vi "udp_vastu.vi"() -> ()   [LabVIEW 2020]
panel:
  out "String":string
  in  "Stop":bool
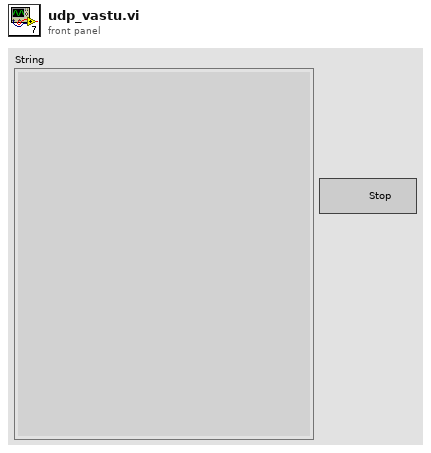
[diagram p1: front panel]
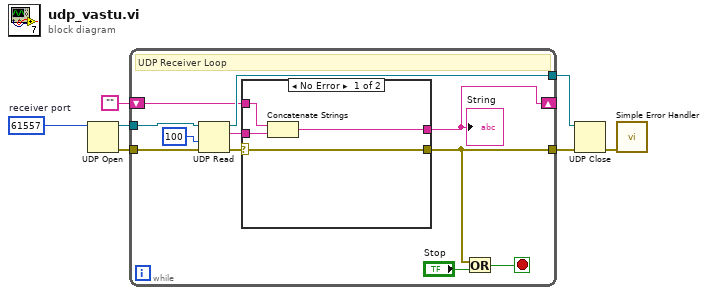
[diagram p0: block diagram]
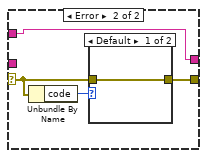
[diagram p2: hidden frame]
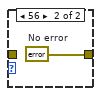
[diagram p3: hidden frame]
diagram:
  w2 = u16 61557  # receiver port
  n1 = UDP Open(11:w2) -> (port=w3:refnum<k16>, 0:w4:errorcluster)  [unwired: 4 in, 1 out]
  n2 = while {
    tunnel: w3 -> [w18]
    tunnel: [w10] -> w7
    tunnel: w4 -> [w15]
    tunnel: [w11] -> w5
    shift-right: [w8] -> _
    shift-left: "" -> [w9]
    stop <- w16 stop-if-true
    # "UDP Receiver Loop"
    n3 = UDP Read(connection ID=w18, timeout ms (25000)=100, 8:w15) -> (data out=w13:string, error out=w12:errorcluster, 3:w10:refnum<k16>)  [unwired: 3 out]
    n4 = case shown="No Error" w12 {
      selector: w12 -> [w22 w25]
      tunnel: w13 -> [w21 _]
      tunnel: [w22 w24] -> w11
      tunnel: w9 -> [w20 w23]
      tunnel: [w19 w23] -> w8
      frame No Error {
        # "Sender sent data. Update chat."
        n5 = Concatenate Strings(w20, w21) -> (w19:string)
      }
      frame Error {
        # "Sender did not send data. Ignore timeout error and keep waiting."
        n6 = Unbundle By Name(w25) -> ("code"=w26:i32)
        n7 = case shown="Default" w26 {
          tunnel: w25 -> [w27 _]
          tunnel: [w27 w28] -> w24
          frame Default {
          }
          frame 56 {
            w28 = errorcluster {"status"=FALSE, "code"=0, "source"=""}  # No error
          }
        }
      }
    }
    "String" <- w8
    n8 = Or(x=w11, y="Stop") -> (x .or. y?=w16:bool)
  }
  n9 = UDP Close(connection ID=w7, 8:w5) -> (error out=w6:errorcluster)  [unwired: 1 out]
  n10 = call <vilib>:"Simple Error Handler.vi"("error in (no error)"=w6) -> ()  [unwired: 1 in, 8 out]
